vi "Get_value_from_string.vi"(2 "Show Dialog?":bool, 3 "Input string":string, 4 "Variable name":string) -> (0 "Status":enum16{"Char in string", "Char not in string"}(ring), 1 "Value":dbl=-999.0 format="%.2f")   [LabVIEW 2010]
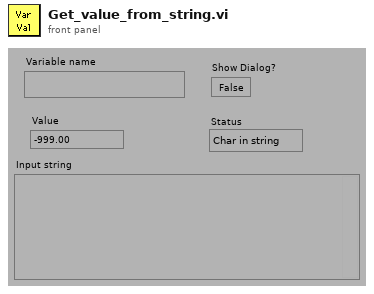
[diagram p1: front panel]
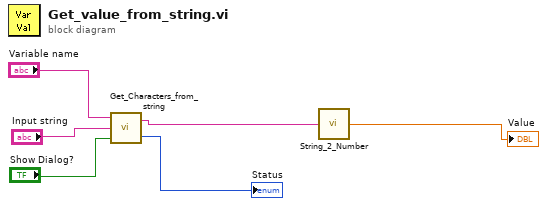
[diagram p0: block diagram]
diagram:
  n1 = call "Get_Characters_from_string.vi"("Show Dialog?"="Show Dialog?", "Input string"="Input string", "Variable name"="Variable name") -> ("Status"=→"Status":enum16{"Char in string", "Char not in string"}, "Value"=w1:string)
  n2 = call "String_2_Number.vi"("Value"=w1) -> ("Numeric"=→"Value":dbl)
